vi "主画面_古田户外.vi"() -> ()   [LabVIEW 2016]
uses:
  <vilib>/Utility/config.llb/Read Key (String).vi
  <vilib>/Utility/config.llb/NI_LVConfig.lvlib
  PLC/PLC.lvlib
  data/FreeMem.dll
panel:
  in  "全屏":T1
  out "站点名称":string="站点名称"
  out "时间显示":string="2017-05-09 10:50:42"
  out "Version":string="Version:1.0.0"
  in  "主画面菜单":enum32{"首页", "数据查询", "运维调试", "系统设置"}(xcontrol)
  # "一体化微 型 水 质 监 测 站"
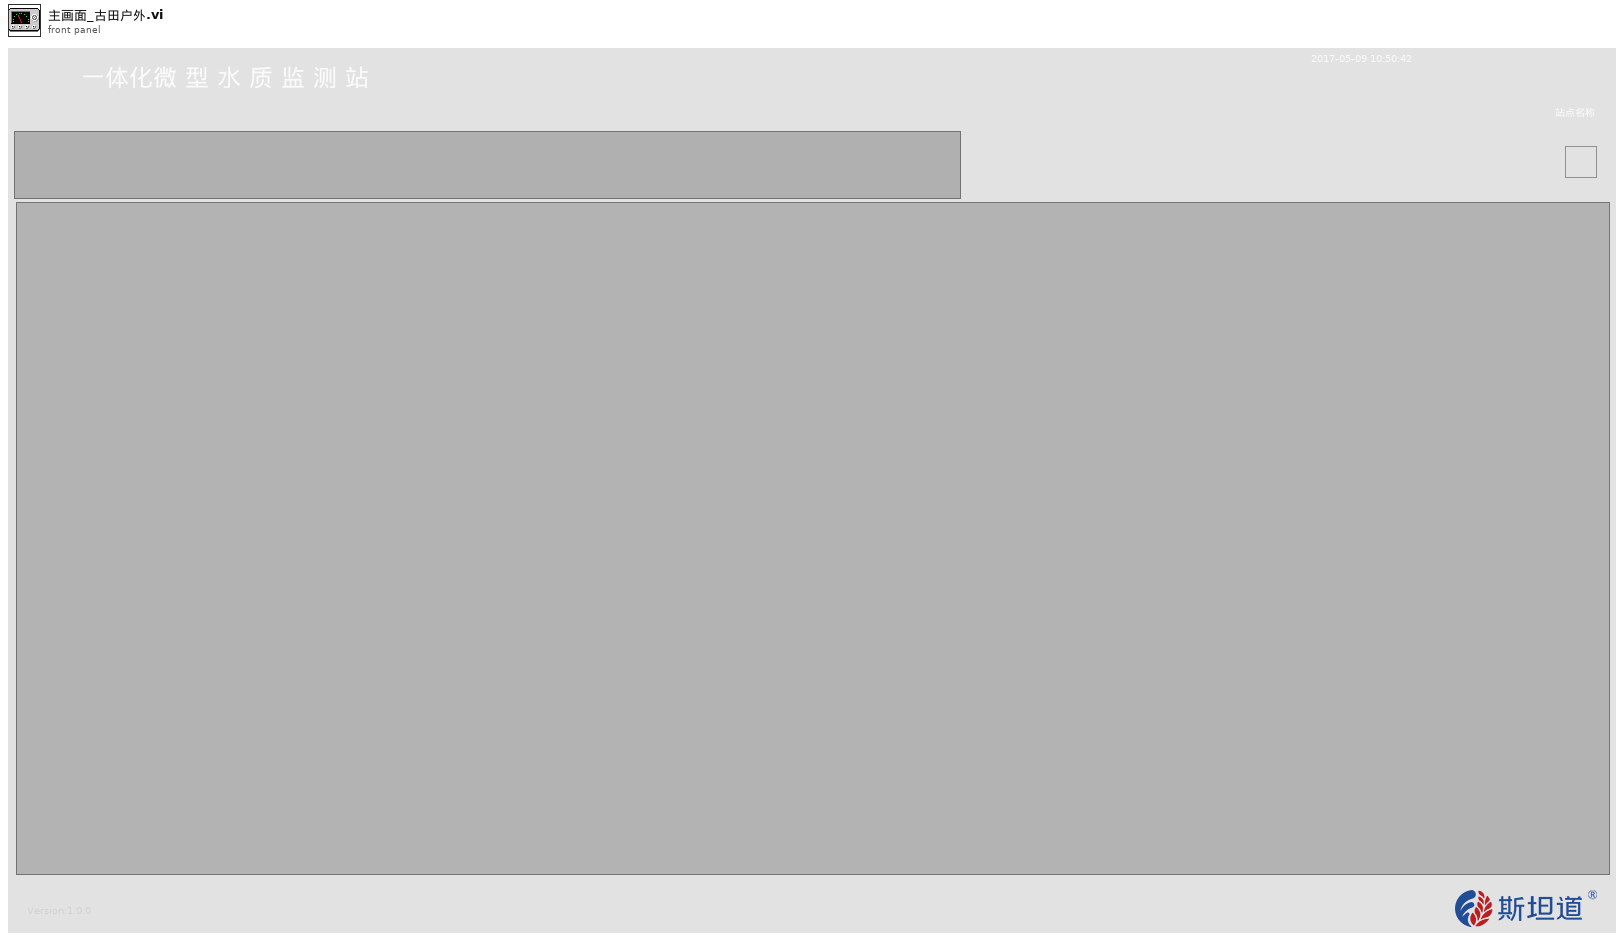
[diagram p1: front panel]
types:
  T1 = typedef "全屏按钮.ctl" = bool
  T2 = cluster{"时间标识":timestamp, "设备":string, "日志信息":string, "流程参数":string}
  T3 = enum32{"invalid app kind", "Development System", "Run Time System", "Student Edition", "Embedded LabVIEW", "Evaluation", "Custom"}
  T4 = typedef "NI_LVConfig.lvlib/Config Data RefNum.ctl" = refnum<k1>
  T5 = cluster{"Y0":bool, "Y1":bool, "Y2":bool, "Y3":bool, "Y4":bool, "Y5":bool, "Y6":bool, "Y7":bool, "Y8":bool, "Y9":bool, "Y10":bool, "Y11":bool, "Y12":bool, "Y13":bool, "Y14":bool, "Y15":bool}
  T6 = enum32{"Bad", "Idle", "Run top level", "Running"}
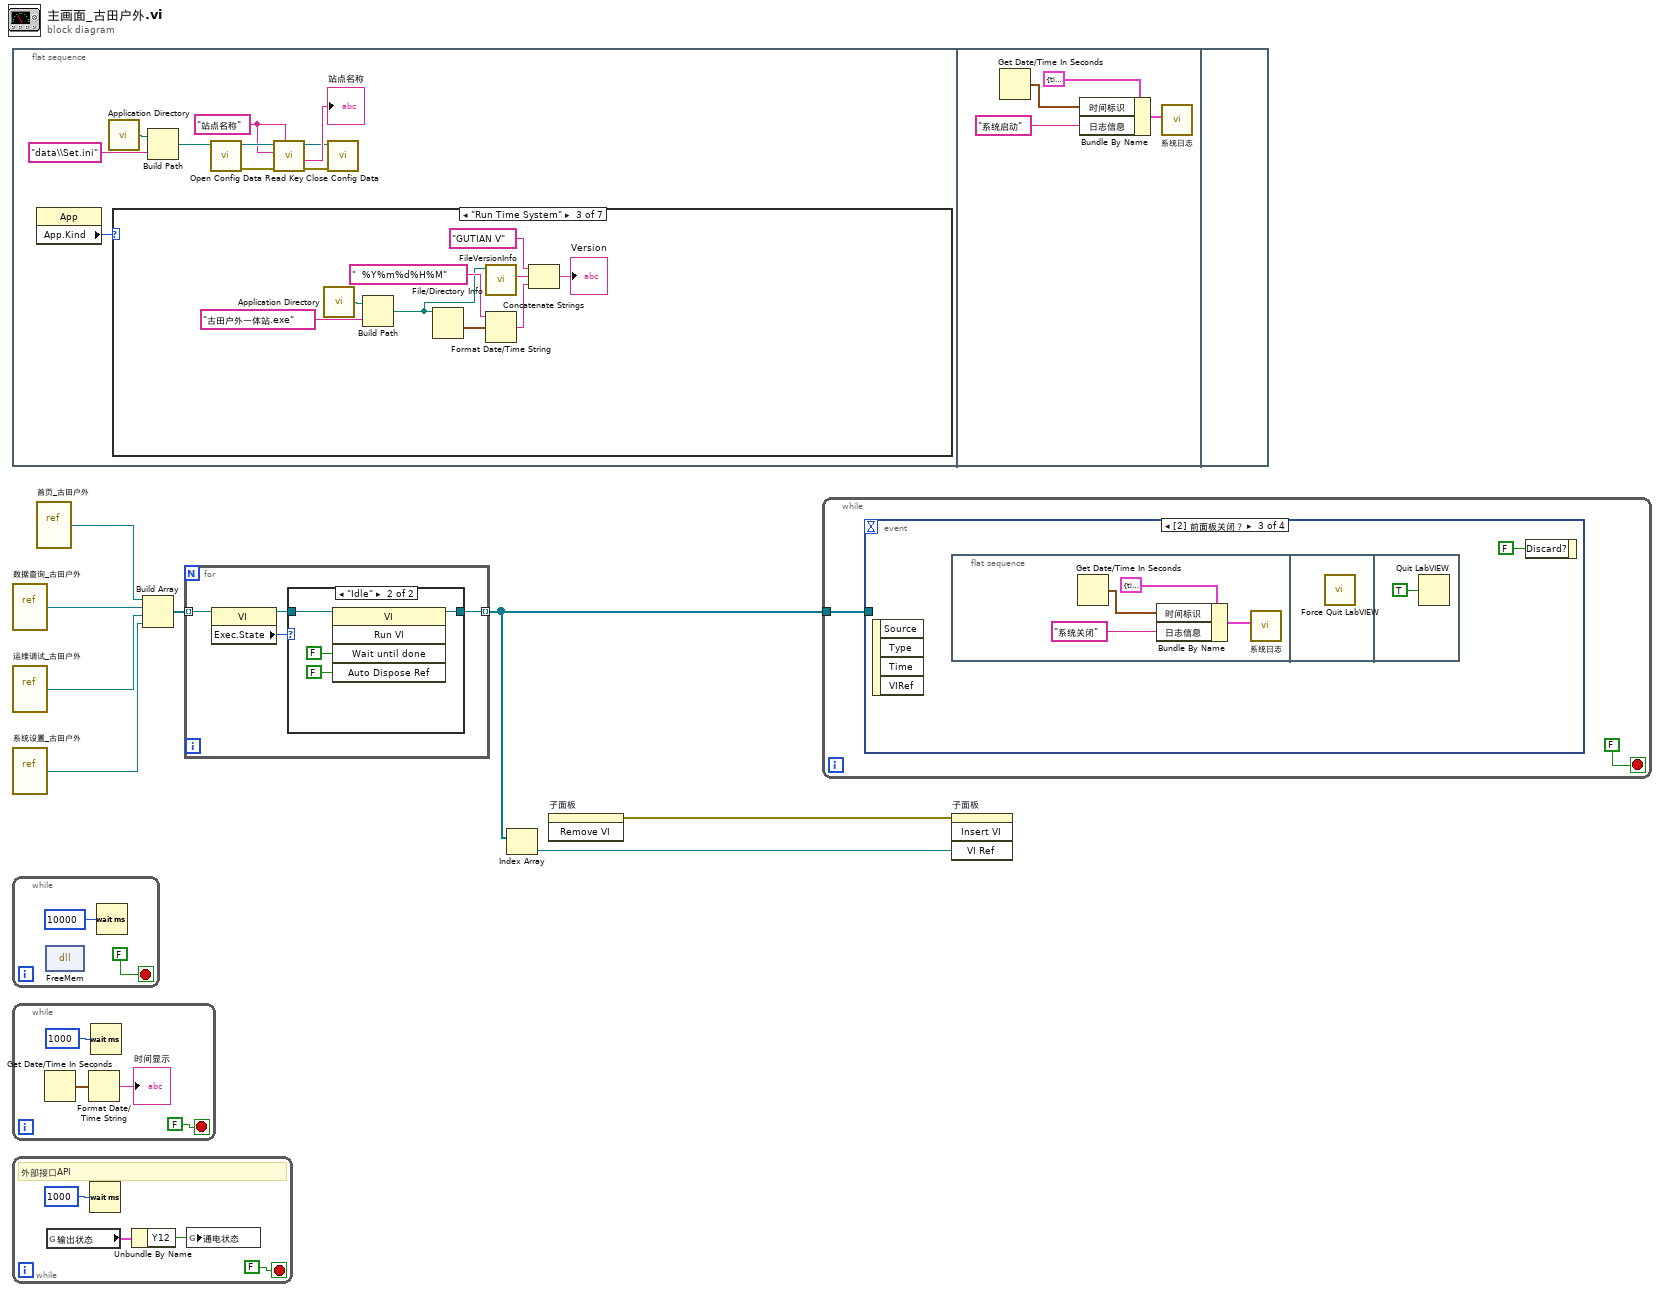
[diagram p0: block diagram]
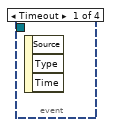
[diagram p9: hidden frame]
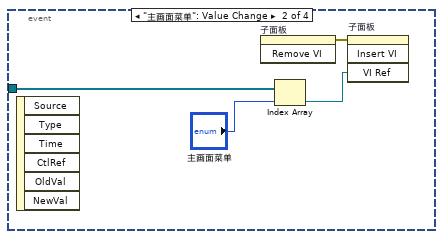
[diagram p10: hidden frame]
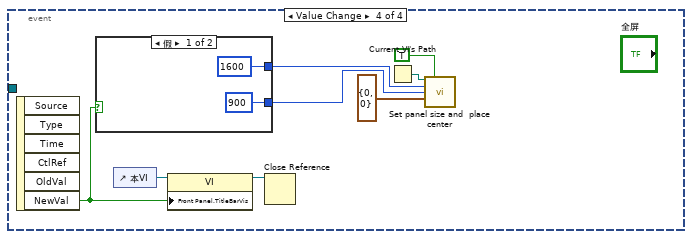
[diagram p11: hidden frame]
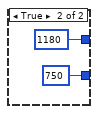
[diagram p12: hidden frame]
diagram:
  n1 = flat-sequence {
    frame #0 {
      w9 = "站点名称" ("section")
      n2 = property class="App"() -> ("App.Kind"=w18:T3)  [unwired: 2 in, 2 out]
      n3 = call <vilib>:"Application Directory.vi"() -> ("Application Directory"=w12:path)
      n4 = case shown="\"Run Time System\"" w18 {
        frame "invalid app kind" {
        }
        frame "Development System", Default {
        }
        frame "Run Time System" {
          n5 = call <vilib>:"Application Directory.vi"() -> ("Application Directory"=w26:path)
          n6 = Build Path(base path=w26, name or relative path="古田户外一体站.exe" ("名称或相对路径")) -> (appended path=w20:path)
          n7 = File/Directory Info(path=w20) -> (last mod=w22:timestamp)  [unwired: 1 in, 6 out]
          n8 = call <vilib>:"FileVersionInfo.vi"("Application Path in"=w20) -> ("File Version Info"=w24:string)  [unwired: 7 in, 3 out]
          n9 = Format Date/Time String(time format string (%c)="  %Y%m%d%H%M" ("时间格式字符串(%c)"), seconds (now)=w22) -> (date/time string=w19:string)  [unwired: 1 in]
          n10 = Concatenate Strings("GUTIAN V" ("字符串"), w24, w19) -> (→"Version":string)
        }
        frame "Student Edition" {
        }
        frame "Embedded LabVIEW" {
        }
        frame "Evaluation" {
        }
        frame "Custom" {
        }
      }
      n11 = Build Path(base path=w12, name or relative path="data\\Set.ini" ("名称或相对路径")) -> (appended path=w10:path)
      n12 = call <vilib>:"Open Config Data.vi"("configuration file path"=w10) -> ("error out"=w14:errorcluster, "refnum"=w17:T4)  [unwired: 8 in, 1 out]
      n13 = call-poly <vilib>:"Read Key.vi"("section"=w9, "error in (no error)"=w14, "key"=w9, "refnum"=w17) -> ("error out"=w13:errorcluster, "value"=→"站点名称":string, "refnum out"=w15:T4)  [unwired: 4 in, 1 out]
      n14 = call <vilib>:"Close Config Data.vi"("error in (no error)"=w13, "refnum"=w15) -> ()  [unwired: 8 in, 2 out]
    }
    frame #1 {
      n15 = Get Date/Time In Seconds() -> (seconds since 1Jan1904=w29:timestamp)
      n16 = Bundle By Name(cluster=T2 {"时间标识"=timestamp(0 s since 1904-01-01), "设备"="系统", "日志信息"="", "流程参数"=""} ("data in"), "时间标识"=w29, "日志信息"="系统启动") -> (w30:T2)
      n17 = call "系统日志.vi"("data in"=w30) -> ()  [unwired: 11 in]
    }
    frame #2 {
    }
  }
  n18 = vi-ref "数据查询_古田户外.vi"() -> (w4:refnum<vi>)
  n19 = vi-ref "运维调试_古田户外.vi"() -> (w3:refnum<vi>)
  n20 = vi-ref "系统设置_古田户外.vi"() -> (w2:refnum<vi>)
  n21 = while {
    stop <- FALSE stop-if-true
    n22 = dll-call lib="PTH2sabs CUsersHsiao\nSynologyDrive工作资料\t待发货古田项目GT一体站项目dataFreeMem.dll" fn="FreeMem"() -> ()  [unwired: 4 in, 2 out]
    n23 = Wait (ms)(milliseconds to wait=u32 10000 ("等待时间（毫秒）")) -> ()  [unwired: 1 out]
  }
  n24 = while {
    stop <- FALSE stop-if-true
    n25 = Get Date/Time In Seconds() -> (seconds since 1Jan1904=w34:timestamp)
    n26 = Format Date/Time String(seconds (now)=w34) -> (date/time string=→"时间显示":string)  [unwired: 2 in]
    n27 = Wait (ms)(milliseconds to wait=u32 1000 ("等待时间（毫秒）")) -> ()  [unwired: 1 out]
  }
  n28 = while "While循环" {
    stop <- FALSE stop-if-true
    # "外部接口API"
    n29 = global read "采配水全局变量.vi" "输出状态"() -> (w41:T5)
    n30 = Wait (ms)(milliseconds to wait=u32 1000 ("等待时间（毫秒）")) -> ()  [unwired: 1 out]
    n31 = Unbundle By Name(w41) -> ("Y12"=w40:bool)
    n32 = global write "多参数全局变量.vi" "通电状态"(w40) -> ()
  }
  n33 = vi-ref "首页_古田户外.vi"() -> (w5:refnum<vi>)
  n34 = Build Array(w5, w4, w3, w2) -> (w1:refnum<vi>[])
  n35 = for {
    tunnel: w1 -> [w45] mode=indexing
    tunnel: [w42] -> w7 mode=indexing
    n36 = property class="VI"(reference=w45) -> (reference out=w43:refnum<vi>, "Exec.State"=w44:T6)  [unwired: 1 in, 1 out]
    n37 = case shown="\"Idle\"" w44 {
      tunnel: w43 -> [w46 w48]
      tunnel: [w46 w47] -> w42
      frame "Bad", Default {
      }
      frame "Idle" {
        n38 = invoke class="VI" method="Run VI"(reference=w48, "Wait until done"=FALSE ("结束前等待"), "Auto Dispose Ref"=FALSE ("自动销毁引用")) -> (reference out=w47:refnum<vi>)  [unwired: 2 in, 4 out]
      }
    }
  }
  n39 = Index Array(array=w7) -> (element=w6:refnum<vi>)  [unwired: 1 in]
  n40 = invoke on="子面板" class="SubPnl" method="Remove VI"() -> (error out=w8:errorcluster)  [unwired: 3 in, 2 out]
  n41 = while {
    tunnel: w7 -> [w51]
    stop <- FALSE stop-if-true
    n42 = event shown="[2] 前面板关闭？" {
      selector: _ -> [_ _ _ _]
      dyn-events: _ -> [_ _ _ _]
      timeout: _ -> [_ _ _ _]
      tunnel: w51 -> [_ w55 _ _]
      event Timeout {
        n43 = event-data() -> ()  [unwired: 1 in, 3 out]
      }
      event "主画面菜单": Value Change {
        n44 = event-data() -> ()  [unwired: 1 in, 6 out]
        n45 = invoke on="子面板" class="SubPnl" method="Remove VI"() -> (error out=w53:errorcluster)  [unwired: 3 in, 2 out]
        n46 = Index Array(array=w55, index="主画面菜单") -> (element=w54:refnum<vi>)
        n47 = invoke on="子面板" class="SubPnl" method="Insert VI"(error in=w53, "VI Ref"=w54) -> ()  [unwired: 2 in, 4 out]
      }
      event Panel Close? {
        n48 = event-data() -> ()  [unwired: 1 in, 4 out]
        n49 = flat-sequence {
          frame #0 {
            n50 = Get Date/Time In Seconds() -> (seconds since 1Jan1904=w60:timestamp)
            n51 = Bundle By Name(cluster=T2 {"时间标识"=timestamp(0 s since 1904-01-01), "设备"="系统", "日志信息"="", "流程参数"=""} ("data in"), "时间标识"=w60, "日志信息"="系统关闭") -> (w59:T2)
            n52 = call "系统日志.vi"("data in"=w59) -> ()  [unwired: 11 in]
          }
          frame #1 {
            n53 = call "Force Quit LabVIEW.vi"() -> ()  [unwired: 10 in, 2 out]
          }
          frame #2 {
            n54 = Quit LabVIEW(quit? (T)=TRUE ("退出？(T)")) -> ()
          }
        }
        n55 = event-data("Discard?"=FALSE ("放弃？")) -> ()  [unwired: 1 in, 1 out]
      }
      event Value Change {
        n56 = event-data() -> ("NewVal"=w65:T1)  [unwired: 1 in, 5 out]
        n57 = case shown="假" w65 {
          tunnel: [1600 ("Panel Width") 1180 ("Panel Width")] -> w64
          tunnel: [900 ("Panel Height") 750 ("Panel Height")] -> w63
          frame False {
          }
          frame True {
          }
        }
        n58 = control-ref of="本VI"() -> (w70:refnum<vi>)
        n59 = property class="VI"(reference=w70, "Front Panel.TitleBarVis"=w65) -> (reference out=w66:refnum<vi>)  [unwired: 1 in, 1 out]
        n60 = Close Reference(reference=w66) -> ()  [unwired: 1 in, 1 out]
        n61 = Current VI's Path() -> (path=w69:path)
        n62 = call "Set panel size and  place center.vi"("Path"=w69, "Close Reference (false)"=TRUE, "Panel Width"=w64, "Panel Height"=w63, "FP.Origin in(H & V)"=cluster{"Horizontal":i16, "Vertical":i16} {"Horizontal"=0, "Vertical"=0}) -> ()  [unwired: 6 in, 5 out]
      }
    }
  }
  n63 = invoke on="子面板" class="SubPnl" method="Insert VI"(error in=w8, "VI Ref"=w6) -> ()  [unwired: 2 in, 4 out]
